vi "RSZVB Get Frequency Conversion.vi"(7 "Port (1)":i32=1, 8 "error in (no error)":errorcluster {"code" format="%.0x"}, 9 "Channel (1)":i32=1, 10 "Measurement Type (0: Receiver)":i32(ring) items=["Receiver", "Source"], 11 "VISA session":refnum<visa-resource-name>) -> (0 "error out":errorcluster {"code" format="%.0x"}, 1 "Numerator":i32, 3 "dup VISA session":refnum<visa-resource-name>, 4 "Sweep Type":i32, 5 "Offset":dbl format="%^.3e", 6 "Denominator":i32)   [LabVIEW 2011]
doc: "This VI queries the receiver frequency or the port-specific source frequency for frequency-converting measurements. The receiver/source frequency is either a range (for frequency sweeps) or a CW frequency (for power, time and CW Mode sweeps). The receiver frequency is valid for all ports. \n\nRemote-control command(s):\n[SENSe<Ch>:]FREQuency:CONVersion:ARBitrary?\nSOURce<Ch>:FREQuency<Pt>:CONVersion:ARBitrary:IFRequency?"
uses:
  _utility/RSZVB Global Data.vi
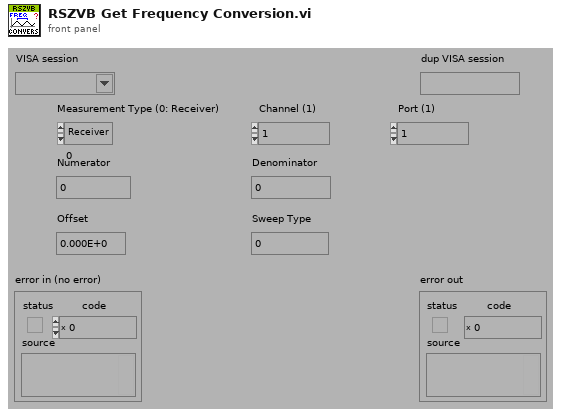
[diagram p1: front panel]
types:
  T1 = cluster{"Error Checking (T: On)":bool, "Installed Options":string[], "Data Valid?":bool, "Ports":i32, "Model":string[], "Option Checking (T: On)":bool}[]
  T2 = cluster{"Error Checking (T: On)":bool, "Installed Options":string[], "Data Valid?":bool, "Ports":i32, "Model":string[], "Option Checking (T: On)":bool}
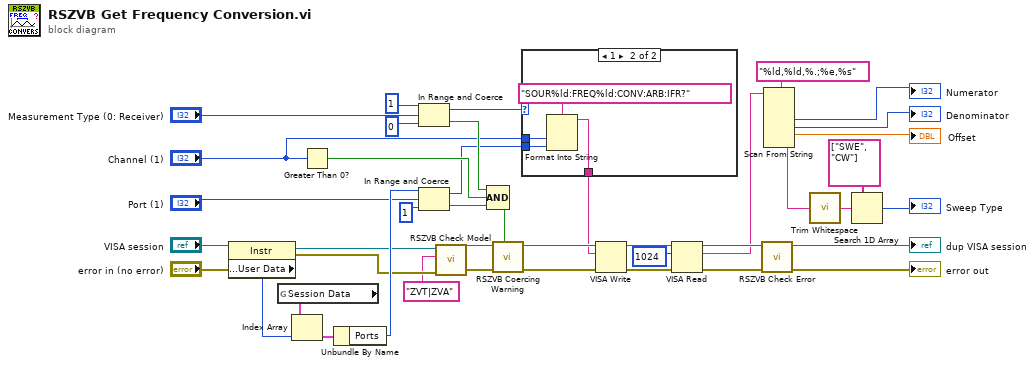
[diagram p0: block diagram]
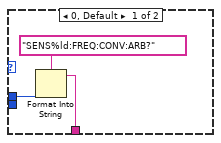
[diagram p2: hidden frame]
diagram:
  n1 = property class="Instr"(reference="VISA session", error in="error in (no error)") -> (reference out=w3:refnum<visa-resource-name>, error out=w2:errorcluster, "General Settings:User Data"=w40:u32)
  n2 = global read "RSZVB Global Data.vi" "Session Data"() -> (w39:T1)
  n3 = Index Array(array=w39, index=w40) -> (element=w38:T2)
  n4 = Greater Than 0?(x="Channel (1)") -> (x > 0?=w28:bool)
  n5 = Unbundle By Name(w38) -> ("Ports"=w36:i32)
  n6 = In Range and Coerce(upper limit=1 ("lower limit"), x="Measurement Type (0: Receiver)", lower limit=0) -> (coerced(x)=w18:i32, In Range?=w29:bool)
  n7 = In Range and Coerce(upper limit=w36, x="Port (1)", lower limit=1) -> (coerced(x)=w14:i32, In Range?=w34:bool)
  n8 = call "RSZVB Check Model.vi"("error in (no error)"=w2, "Model"="ZVT|ZVA" ("Options"), "VISA session"=w3) -> ("error out"=w5:errorcluster, "dup VISA session"=w4:refnum<visa-resource-name>)  [unwired: 7 in]
  n9 = Compound Arithmetic op=AND(w29, w28, w34) -> (w37:bool)
  n10 = call "RSZVB Coercing Warning.vi"("In Range?"=w37, "error in (no error)"=w5, "VISA session"=w4) -> ("error out"=w27:errorcluster, "dup VISA session"=w26:refnum<visa-resource-name>)  [unwired: 7 in]
  n11 = case shown="1" w18 {
    tunnel: [w45 w48] -> w19
    tunnel: "Channel (1)" -> [w44 w47]
    tunnel: w14 -> [_ w46]
    frame 0, Default {
      n12 = Format Into String(format string="SENS%ld:FREQ:CONV:ARB?", w44) -> (resulting string=w45:string)  [unwired: 2 in, 1 out]
    }
    frame 1 {
      n13 = Format Into String(format string="SOUR%ld:FREQ%ld:CONV:ARB:IFR?", w47, w46) -> (resulting string=w48:string)  [unwired: 2 in, 1 out]
    }
  }
  n14 = VISA Write(VISA resource name=w26, write buffer=w19, error in (no error)=w27) -> (VISA resource name out=w20:refnum<visa-resource-name>, error out=w21:errorcluster)  [unwired: 1 out]
  n15 = VISA Read(VISA resource name=w20, byte count=u32 1024 ("byte count (0)"), error in (no error)=w21) -> (VISA resource name out=w24:refnum<visa-resource-name>, read buffer=w6:string, error out=w23:errorcluster)  [unwired: 1 out]
  n16 = call "RSZVB Check Error.vi"("error in (no error)"=w23, "VISA session"=w24) -> ("error out"=→"error out":errorcluster, "dup VISA session"=→"dup VISA session":refnum<visa-resource-name>)  [unwired: 8 in]
  n17 = Scan From String(format string="%ld,%ld,%.;%e,%s", input string=w6) -> (output 1=→"Numerator":i32, output 2=→"Denominator":i32, output 3=→"Offset":dbl, output 4=w8:string)  [unwired: 6 in, 3 out]
  n18 = call <vilib>:"Trim Whitespace.vi"("string"=w8) -> ("trimmed string"=w9:string)  [unwired: 1 in]
  n19 = Search 1D Array(1D array=string[] ["SWE", "CW"] ("array 2"), element=w9) -> (index of element=→"Sweep Type":i32)  [unwired: 1 in]
